vi "epoll_wait.vi"(8 "error in":errorcluster, 10 "timeout ms":i32=-1, 11 "epoll in":refnum<class "epoll.lvclass">) -> (0 "error out":errorcluster, 2 "timed out":bool, 3 "epoll out":refnum<class "epoll.lvclass">)   [LabVIEW 2020, in "PCANBasic.lvlib" / "epoll.lvclass"]
uses:
  epoll.lvclass
  epoll.lvclass/epoll.ctl
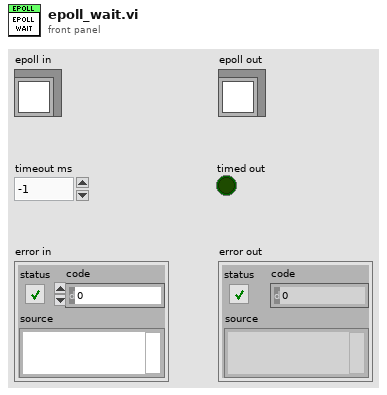
[diagram p1: front panel]
types:
  T1 = enum16{"unspecified", "close", "epoll_create", "epoll_ctl", "epoll_wait"}
  T2 = enum16{"NO ERROR", "EPERM", "ENOENT", "ESRCH", "EINTR", "EIO", "ENXIO", "E2BIG", "ENOEXEC", "EBADF", "ECHILD", "EAGAIN", "ENOMEM", "EACCES", "EFAULT", "ENOTBLK", "EBUSY", "EEXIST", "EXDEV", "ENODEV", "ENOTDIR", "EISDIR", "EINVAL", "ENFILE", "EMFILE", "ENOTTY", "ETXTBSY", "EFBIG", "ENOSPC", "ESPIPE", "EROFS", "EMLINK", "EPIPE", "EDOM", "ERANGE", "EDADLK", "ENAMETOOLONG", "ENOLCK", "ENOSYS", "ENOTEMPTY", "ELOOP", "EWOULDBLOCK", "ENOMSG", "EIDRM", "ECHRNG", "EL2NSYNC", "EL3HLT", "EL3RST", "ELNRNG", "EUNATCH", "ENOCSI", "EL2HLT", "EBADE", "EBADR", "EXFULL", "ENOANO", "EBADRQC", "EBADSLT", "EDEADLOCK", "EBFONT", "ENOSTR", "ENODATA", "ETIME", "ENOSR", "ENONET", "ENOPKG", "EREMOTE", "ENOLINK", "EADV", "ESRMNT", "ECOMM", "EPROTO", "EMULTIHOP", "EDOTDOT", "EBADMSG", "EOVERFLOW", "ENOTUNIQ", "EBADFD", "EREMCHG", "ELIBACC", "ELIBBAD", "ELIBSCN", "ELIBMAX", "ELIBEXEC", "ELISEQ", "ERESTART", "ESTRPIPE", "EUSERS", "ENOTSOCK", "EDESTADDRREQ", "EMSGSIZE", "EPROTOTYPE", "ENOPROTOOPT", "EPROTONOSUPPORT", "ESOCKTNOSUPPORT", "EOPNOTSUPP", "EPFNOSUPPORT", "EAFNOSUPPORT", "EADDRINUSE", "EADDRNOTAVAIL", "ENETDOWN", "ENETUNREACH", "ENETRESET", "ECONNABORTED", "ECONNRESET", "ENOBUFS", "EISCONN", "ENOTCONN", "ESHUTDOWN", "ETOOMANYREFS", "ETIMEDOUT", "ECONNREFUSED", "EHOSTDOWN", "EHOSTUNREACH", "EALREADY", "EINPROGRESS", "ESTALE", "EUCLEAN", "ENOTNAM", "ENAVAIL", "EISNAM", "EREMOTEIO", "EDQUOT", "ENOMEDIUM", "EMEDIUMTYPE", "ECANCELED", "ENOKEY", "EKEYEXPIRED", "EKEYREVOKED", "EKEYREJECTED", "EOWNERDEAD", "ENOTRECOVERABLE", "ERFKILL", "EHWPOISON", "UNDEFINED"}
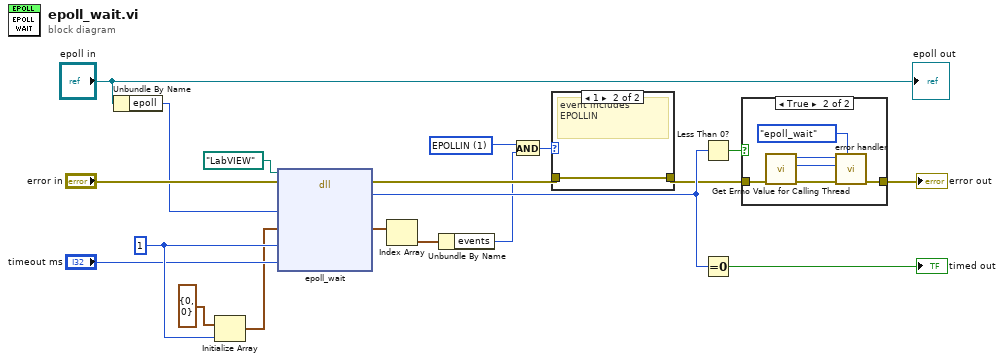
[diagram p0: block diagram]
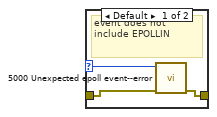
[diagram p2: hidden frame]
diagram:
  w5 = u32 1 items=["EPOLLIN"=1, "EPOLLPRI"=2, "EPOLLOUT"=4, "EPOLLERR"=8, "EPOLLHUP"=16, "EPOLLRDNORM"=64, "EPOLLRDBAND"=128, "EPOLLWRNORM"=256, "EPOLLWRBAND"=512, "EPOLLMSG"=1024, "EPOLLRDHUP"=8192, "EPOLLWAKEUP"=536870912, "EPOLLONESHOT"=1073741824, "EPOLLET"=2147483648] ("event")
  w14 = u32 1 ("max events")
  n1 = Unbundle By Name("epoll in") -> ("epoll"=w7:i32)
  n2 = Initialize Array(cluster{"events":u32, "data":u64} {"events"=0, "data"=0} ("event"), w14) -> (w10:cluster{"events":u32, "data":u64}[])
  n3 = dll-call lib="LabVIEW" fn="epoll_wait"(path in=path "LabVIEW", error in="error in", "epfd"=w7, "event"=w10, "max_events"=w14, "timeout"="timeout ms") -> (error out=w18:errorcluster, "return"=w12:i32, "event"=w9:cluster{"events":u32, "data":u64}[])  [unwired: 4 in, 1 out]
  n4 = Index Array(array=w9) -> (element=w4:cluster{"events":u32, "data":u64})  [unwired: 1 in]
  n5 = Unbundle By Name(w4) -> ("events"=w3:u32)
  n6 = And(x=w5, y=w3) -> (x .and. y?=w1:u32)
  n7 = case shown="1" w1 {
    selector: w1 -> [w20 _]
    tunnel: w18 -> [w22 w23]
    tunnel: [w21 w23] -> w2
    frame Default {
      # "event does not\ninclude EPOLLIN"
      n8 = call "5000 Unexpected epoll event--error.vi"("error in"=w22, "Event"=w20) -> ("error out"=w21:errorcluster)  [unwired: 8 in, 1 out]
    }
    frame 1 {
      # "event includes\nEPOLLIN"
    }
  }
  n9 = Less Than 0?(x=w12) -> (x < 0?=w16:bool)
  n10 = Equal To 0?(x=w12) -> (x = 0?=→"timed out":bool)
  n11 = case shown="True" w16 {
    tunnel: w2 -> [w24 w30]
    tunnel: [w24 w29] -> w17
    frame False {
    }
    frame True {
      n12 = call "Get Errno Value for Calling Thread.vi"("error in"=w30) -> ("error out"=w28:errorcluster, "errno number"=w26:i32, "errno"=w27:T2)  [unwired: 8 in]
      n13 = call "error handler.vi"("function (unspecified)"=T1."epoll_wait", "error in"=w28, "errno number"=w26, "errno"=w27) -> ("error out"=w29:errorcluster)  [unwired: 7 in]
    }
  }
  "error out" <- w17
  "epoll out" <- "epoll in"
